vi "CALC_PAR_DEL_NAME_M.vi"(0 "VISA IN":refnum<visa-resource-name>, 1 "Measurement Name":string, 5 "error in":errorcluster, 7 "Channel":i32) -> (14 "VISA Out":refnum<visa-resource-name>, 19 "error out":errorcluster)   [LabVIEW 2018, in "PNA-X.lvlib"]
doc: "CALCulate<cnum>:PARameter:DELete[:NAME] <Mname> \n(Write-only) Deletes the specified measurement. \nSee Critical Note \nParameters \n<cnum> Channel number of the measurement. There must be a selected measurement \non that channel. If unspecified, <cnum> is set to 1. \n<Mname> String - Name of the measurement \nExamples CALC:PAR:DEL 'TEST' \ncalculate2:parameter:delete 'test' \nQuery Syntax Not Applicable \nDefault Not Applicable \nCALCulate:PARameter:DELete:ALL \n1557\n\n(Write-only) Deletes all measurements on the PNA. \nSee Critical Note \nParameters \nExamples CALC:PAR:DEL:ALL \nQuery Syntax Not Applicable \nDefault Not Applicable"
uses:
  PNA-X.lvlib
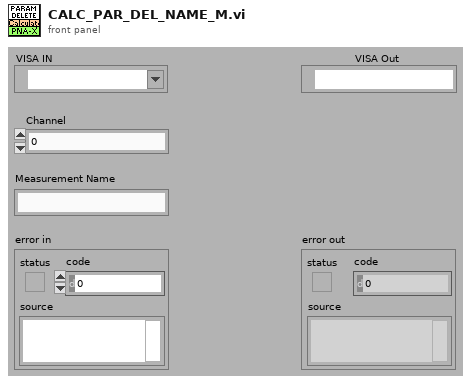
[diagram p1: front panel]
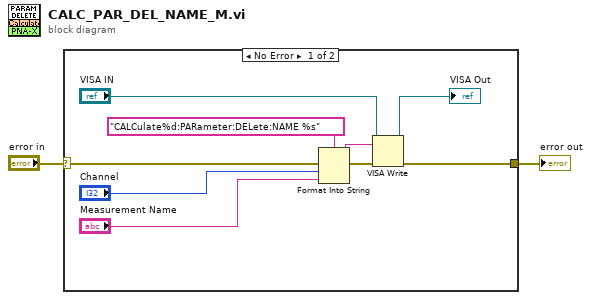
[diagram p0: block diagram]
diagram:
  n1 = case shown="No Error" "error in" {
    selector: "error in" -> [w11 w12]
    tunnel: [w6 w12] -> w1
    frame No Error {
      n2 = Format Into String(format string="CALCulate%d:PARameter:DELete:NAME %s" ("Cmdline"), error in=w11, "Channel", "Measurement Name") -> (resulting string=w9:string, error out=w10:errorcluster)  [unwired: 1 in]
      n3 = VISA Write(VISA resource name="VISA IN", write buffer=w9, error in (no error)=w10) -> (VISA resource name out=→"VISA Out":refnum<visa-resource-name>, error out=w6:errorcluster)  [unwired: 1 out]
    }
    frame Error {
    }
  }
  "error out" <- w1
